vi "LIDAR Debug Platform.vi"() -> ()   [LabVIEW 2010]
uses:
  <vilib>/userDefined/High Color/nirio_resource_hc.ctl
  <vilib>/rvi/interface/nirviOpenFPGA/nirviOpenFPGA.xnode
  FPGA Bitfiles/Athena Brain.lvproj_FPGA Target 2_serial FPGA Main.vi.lvbitx
  serial FPGA Main.vi
  <vilib>/rvi/interface/nirviMethod/nirviMethod.xnode
  <vilib>/rvi/DataTransferAndStorage/Container/XNode/niFpgaContainer.xnode
  Unsorted Files from Athena/behaviors/driveable path/drivable paths global.vi
  serial FPGA main reference type def.ctl
panel:
  out "process time":u32
  out "transform":u32
  out "XY Graph":T1(graph)
  in  "write?":bool
  in  "Data to write":string="\u0002\u0000\u0002\u0000 $4\b"
  out "error out":errorcluster
  out "LIDAR String":string
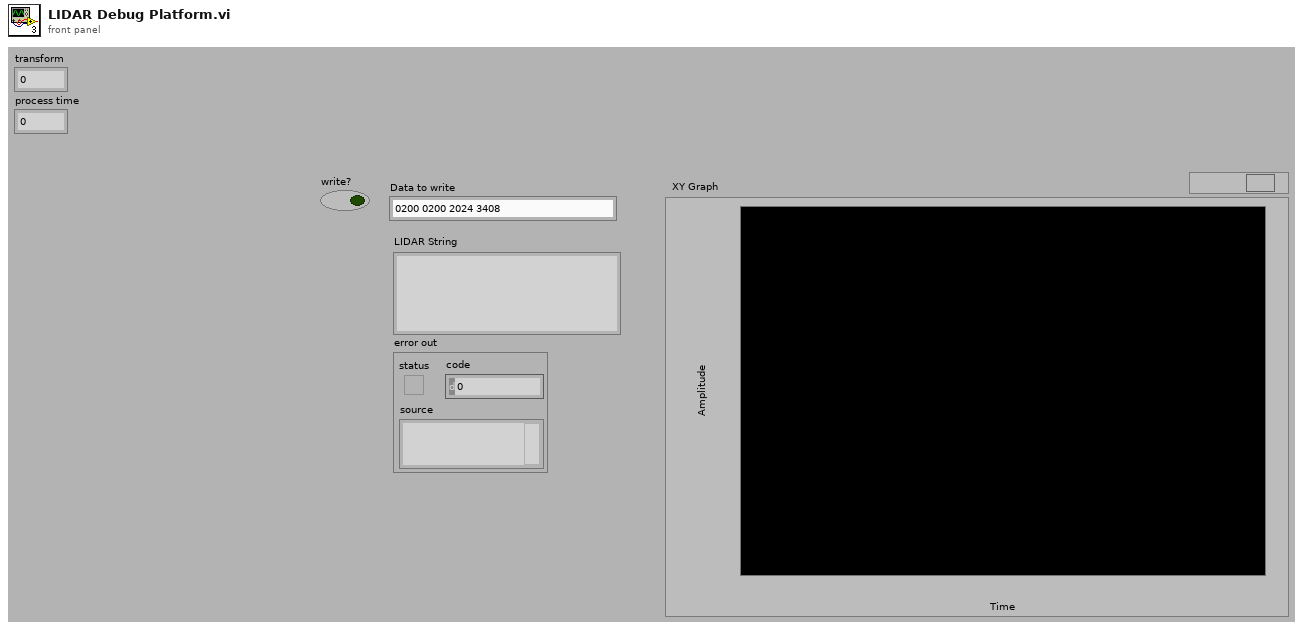
[diagram p1: front panel]
types:
  T1 = cluster{"New X Position":i16, "New Y Position":i16}[]
  T2 = typedef "serial FPGA main reference type def.ctl" = refnum<k20>
  T3 = enum16{"confirm check sum", "check status byte", "read measured values", "confirm measurement", "confirm command", "read message length", "read address", "wait for \"02\""}
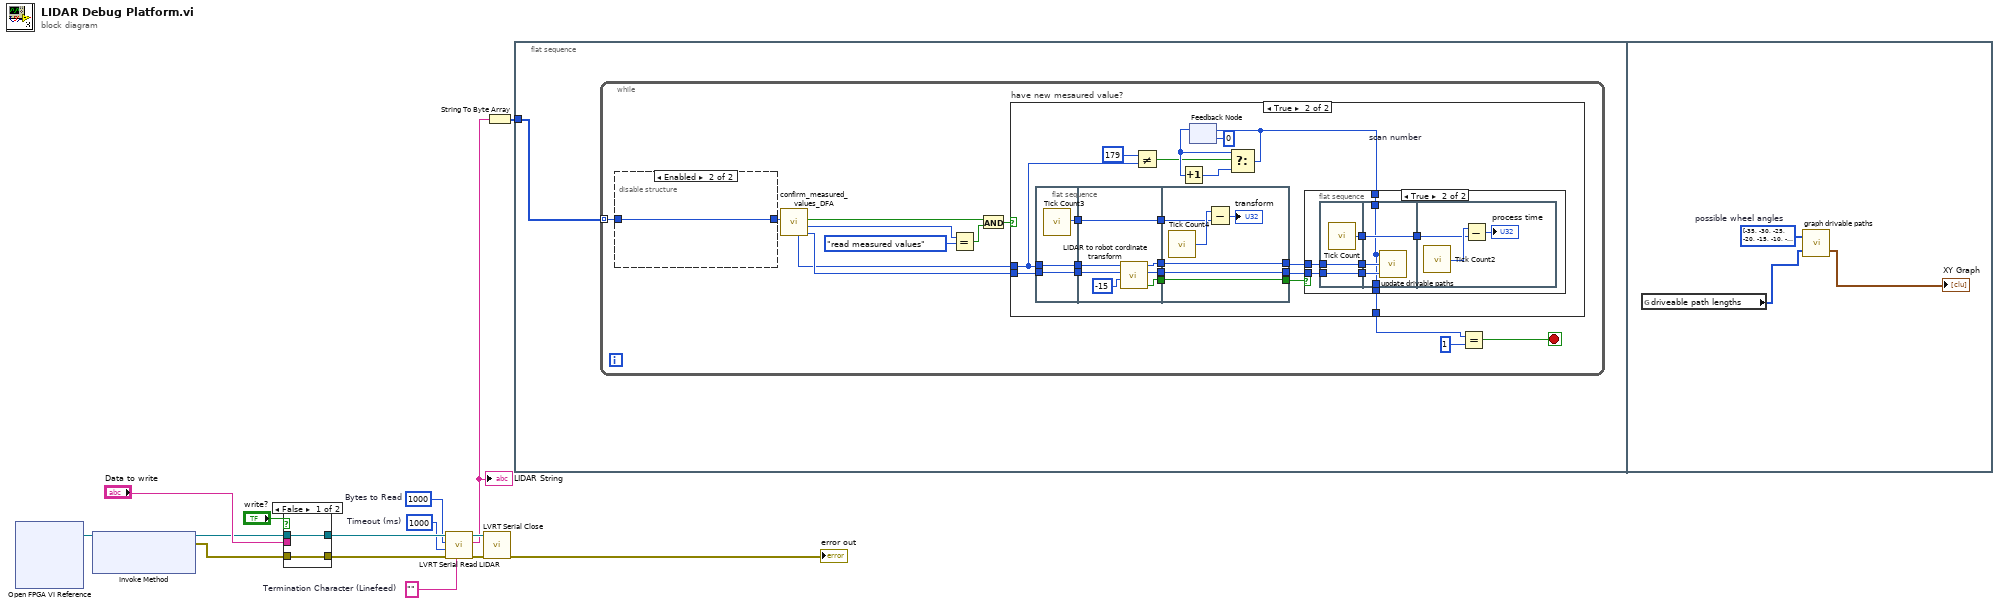
[diagram p0: block diagram]
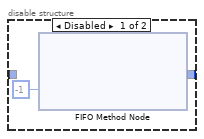
[diagram p2: hidden frame]
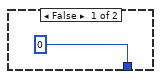
[diagram p3: hidden frame]
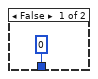
[diagram p4: hidden frame]
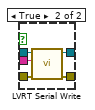
[diagram p5: hidden frame]
diagram:
  w5 = ""  # Termination Character (Linefeed)
  w10 = 1000  # Timeout (ms)
  w12 = u32 1000  # Bytes to Read
  n1 = xnode "Open FPGA VI Reference"() -> ("FPGA VI Reference Out"=w8:T2)  [unwired: 2 in, 1 out]
  n2 = xnode "Invoke Method"("FPGA VI Reference In"=w8) -> ("FPGA VI Reference Out"=w7:T2, "error out"=w6:errorcluster)  [unwired: 1 in, 1 out]
  n3 = case shown="False" "write?" {
    tunnel: "Data to write" -> [_ w22]
    tunnel: [w16 w21] -> w14
    tunnel: [w17 w20] -> w13
    tunnel: w7 -> [w17 w19]
    tunnel: w6 -> [w16 w18]
    frame False {
    }
    frame True {
      n4 = call "LVRT Serial Write.vi"("error in (no error)"=w18, "String"=w22, "FPGA Main Ref"=w19) -> ("error out"=w21:errorcluster, "FPGA Main Ref Out"=w20:T2)  [unwired: 7 in]
    }
  }
  n5 = call "LVRT Serial Read LIDAR.vi"("Termination Character (Linefeed)"=w5, "error in (no error)"=w14, "Timeout (ms) (-1: no timeout)"=w10, "Bytes to Read"=w12, "FPGA Main Ref"=w13) -> ("error out"=w4:errorcluster, "LIDAR"=w2:string, "FPGA Main Ref Out"=w3:T2)  [unwired: 4 in]
  "LIDAR String" <- w2
  n6 = call "LVRT Serial Close.vi"("error out"=w4, "FPGA Main Ref"=w3) -> ("error out"=→"error out":errorcluster)  [unwired: 9 out]
  n7 = String To Byte Array(string=w2) -> (unsigned byte array=w1:u8[])
  n8 = flat-sequence {
    tunnel: w1 -> [w23]
    frame #0 {
      n9 = while {
        tunnel: w23 -> [w28] mode=indexing
        stop <- w24 stop-if-true
        n10 = disable-structure shown="Enabled" {
          disable-tunnel: [w37 w38] -> w35
          disable-tunnel: w28 -> [_ w38]
          frame Disabled {
            n11 = xnode ("FIFO Method Node")("Timeout"=-1) -> ("Element"=w37)  [unwired: 1 in, 2 out]
          }
          frame Enabled {
          }
        }
        n12 = call "confirm_measured_values_DFA.vi"("LIDAR raw data"=w35) -> ("last measured value"=w34:u16, "parser state"=w33:T3, "new value?"=w32:bool, "angle"=w26:u8)  [unwired: 7 in]
        n13 = Equal?(x=w33, y=T3."read measured values" ("parser state")) -> (x = y?=w29:bool)
        n14 = And(x=w32, y=w29) -> (x .and. y?=w31:bool)
        n15 = case "have new mesaured value?" shown="True" w31 {
          tunnel: w34 -> [_ w58]
          tunnel: w26 -> [_ w44]
          tunnel: [u8 0 ("y") w40] -> w25
          frame False {
          }
          frame True {
            n16 = flat-sequence {
              tunnel: w44 -> [w79]
              tunnel: w58 -> [w80]
              tunnel: [w80] -> w54
              tunnel: [w79] -> w53
              tunnel: [w78] -> w49
              tunnel: w54 -> [w87]
              tunnel: w53 -> [w83]
              tunnel: [w85] -> w52
              tunnel: [w84] -> w51
              tunnel: [w82] -> w50
              tunnel: w49 -> [w81]
              tunnel: [w81] -> w48
              tunnel: [w91] -> w55
              tunnel: [w92] -> w56
              tunnel: [w93] -> w57
              tunnel: w52 -> [w93]
              tunnel: w51 -> [w92]
              tunnel: w50 -> [w91]
              tunnel: w48 -> [w89]
              frame #0 {
                n17 = call "Tick Count3"() -> ("Tick Count(Ticks)"=w78:u32)
              }
              frame #1 {
                n18 = call "LIDAR to robot cordinate transform.vi"("Lidar Vertical Position"=i8 -15, "Lidar Distance"=w87, "Lidar Scan Angle"=w83) -> ("Is object?"=w82:bool, "Robot Y"=w84:i16, "Lidar X = Robot X"=w85:i16)  [unwired: 3 in, 3 out]
              }
              frame #2 {
                n19 = call "Tick Count4"() -> ("Tick Count(Ticks)"=w90:u32)
                n20 = Subtract(x=w90, y=w89) -> (x-y=→"transform":u32)
              }
            }
            n21 = Not Equal?(x=u8 179, y=w44) -> (x != y?=w45:bool)
            n22 = feedback #1 "scan number"(u8 0 ("y")) -> (w47:u8)
            n23 = Increment(x=w47) -> (x+1=w46:u8)
            n24 = Select(t=w47, s=w45, f=w46) -> (s? t:f=w42:u8)
            n25 = feedback-in #1(w42) -> ()
            n26 = case shown="True" w55 {
              tunnel: w57 -> [_ w67]
              tunnel: w56 -> [_ w66]
              tunnel: w42 -> [_ w61]
              tunnel: [u8 0 ("y") w60] -> w40
              frame False {
              }
              frame True {
                n27 = flat-sequence {
                  tunnel: w66 -> [w69]
                  tunnel: w67 -> [w70]
                  tunnel: [w70] -> w65
                  tunnel: [w69] -> w64
                  tunnel: [w68] -> w63
                  tunnel: w65 -> [w74]
                  tunnel: w64 -> [w73]
                  tunnel: w63 -> [w72]
                  tunnel: [w72] -> w62
                  tunnel: w61 -> [w71]
                  tunnel: [w71] -> w60
                  tunnel: w62 -> [w76]
                  frame #0 {
                    n28 = call "Tick Count"() -> ("Tick Count(Ticks)"=w68:u32)
                  }
                  frame #1 {
                    n29 = call "update drivable paths.vi"("Robot Y"=w73, "Robot X"=w74, "Scan Number"=w71) -> ()  [unwired: 3 in]
                  }
                  frame #2 {
                    n30 = call "Tick Count2"() -> ("Tick Count(Ticks)"=w77:u32)
                    n31 = Subtract(x=w77, y=w76) -> (x-y=→"process time":u32)
                  }
                }
              }
            }
          }
        }
        n32 = Equal?(x=w25, y=u8 1) -> (x = y?=w24:bool)
      }
    }
    frame #1 {
      w96 = i8[] [-35, -30, -25, -20, -15, -10, -5, -1, 1, 5, 10, 15, 20, 25, 30, 35]  # possible wheel angles
      n33 = global read "drivable paths global.vi" "driveable path lengths"() -> (w94:u16[])
      n34 = call "graph drivable paths.vi"("updated max path lengths"=w94, "possible wheel angles"=w96) -> ("XY Graph"=→"XY Graph":T1)  [unwired: 1 in]
    }
  }
